vi "SER_RAND.vi"() -> ()   [LabVIEW 2018]
uses:
  Var_serrure.vi
panel:
  out "Numeric":dbl
  in  "?":bool
  out "LED ROUGE":bool
  out "LED VERTE":bool
  in  "Nr3":dbl(knob) min=0.0 max=9.0 step=1.0 scale=0.0..9.0
  in  "Nr2":dbl(knob) min=0.0 max=9.0 step=1.0 scale=0.0..9.0
  in  "Nr1":dbl(knob) min=0.0 max=9.0 step=1.0 scale=0.0..9.0
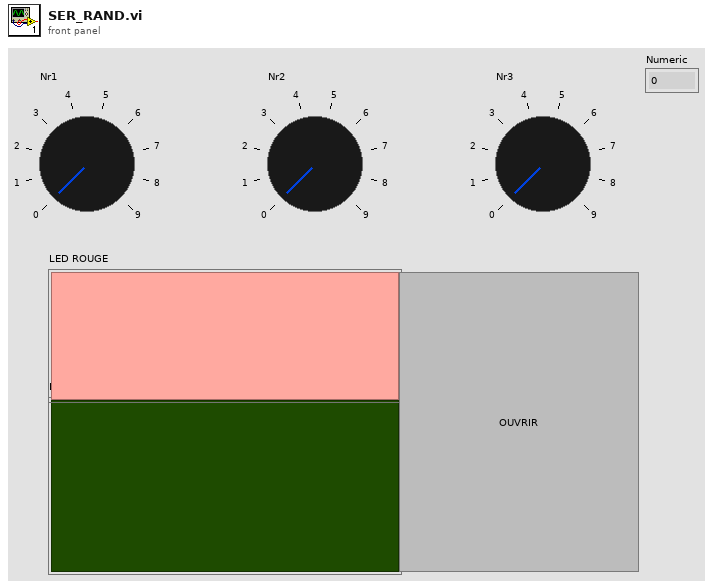
[diagram p1: front panel]
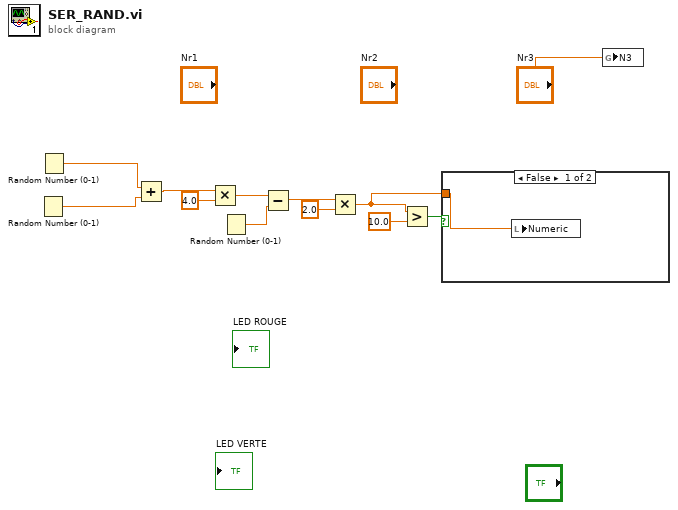
[diagram p0: block diagram]
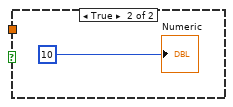
[diagram p2: hidden frame]
diagram:
  n1 = Random Number (0-1)() -> (number: 0 to 1=w11:dbl)
  n2 = Random Number (0-1)() -> (number: 0 to 1=w12:dbl)
  n3 = Add(x=w12, y=w11) -> (x+y=w10:dbl)
  n4 = Multiply(x=w10, y=4.0) -> (x*y=w8:dbl)
  n5 = Random Number (0-1)() -> (number: 0 to 1=w7:dbl)
  n6 = Subtract(x=w8, y=w7) -> (x-y=w5:dbl)
  n7 = Multiply(x=w5, y=2.0) -> (x*y=w1:dbl)
  n8 = Greater?(x=w1, y=10.0) -> (0:w2:bool)
  n9 = case shown="False" w2 {
    tunnel: w1 -> [w13 _]
    frame False {
      n10 = local write "Numeric"(w13) -> ()
    }
    frame True {
      "Numeric" <- 10
    }
  }
  n11 = global write "Var_serrure.vi" "N3"("Nr3") -> ()
